vi "Read Cable Length.vi"(8 "error in (no error)":errorcluster, 11 "Agilent 428x in":refnum<class "Agilent 428x.lvclass">) -> (0 "error out":errorcluster, 2 "Cable Length (0: 0 m)":u32(ring)=1 items=["0 m", "1 m", "2 m", "3 m", "4 m"], 3 "Agilent 428x out":refnum<class "Agilent 428x.lvclass">)   [LabVIEW 2020, in "Agilent 428x.lvclass"]
uses:
  Agilent 428x.lvclass
  Agilent 428x.lvclass/Agilent 428x.ctl
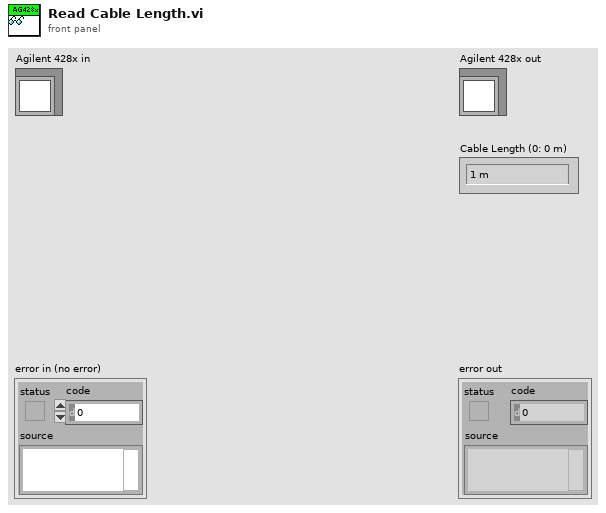
[diagram p1: front panel]
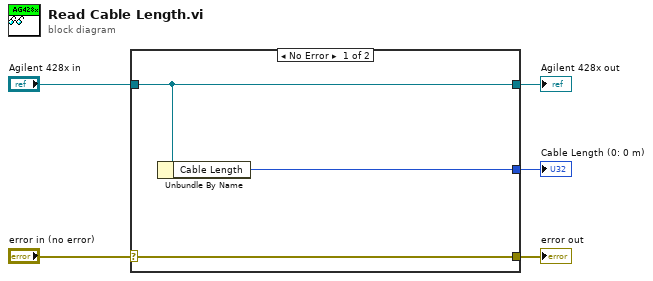
[diagram p0: block diagram]
diagram:
  n1 = case shown="No Error" "error in (no error)" {
    selector: "error in (no error)" -> [w8 w9]
    tunnel: [w8 w9] -> w4
    tunnel: [w7 w10] -> w2
    tunnel: "Agilent 428x in" -> [w7 w10]
    tunnel: [w6 _] -> w1
    frame No Error {
      n2 = Unbundle By Name(w7) -> ("Cable Length"=w6:u32)
    }
    frame Error {
    }
  }
  "error out" <- w4
  "Agilent 428x out" <- w2
  "Cable Length (0: 0 m)" <- w1
